vi "washinglogin.vi"() -> ()   [LabVIEW 2024]
uses:
  <vilib>/Utility/file.llb/Write Delimited Spreadsheet (string).vi
panel:
  in  "stop 9":bool
  in  "stop 4":bool
  out "bytes written 6":i32
  out "bytes written 5":i32
  in  "?":T1(tab)
  out "Validation":string
  in  "Edit":bool
  out "Boolean":bool
  in  "Delete":bool
  in  "Add":bool
  in  "Login":bool
  in  "Password":string
  in  "Username":string
  in  "?":bool
  in  "?":bool
  out "?":dbl(slide) scale=20.0..60.0
  out "?":dbl(slide) scale=20.0..60.0
  in  "?":enum16{"Soak", "Wash", "Rinse", "Spin"}(ring)
  in  "?":enum16{"Hot", "Default", "Cold"}(ring)
  in  "?":bool
  in  "?":enum16{"High", "Medium", "Low"}(ring)
  out "ON led":bool
  in  "?":bool
  out "?":dbl
  in  "?":dbl min=0.0 max=9999.0
  in  "?":string
  out "?":dbl
  in  "?":string
  in  "?":dbl min=0.0 max=9999.0
  in  "?":enum16{"Soak", "Wash", "Rinse", "Spin"}(ring)
  in  "?":bool
  in  "?":enum16{"High", "Medium", "Low"}(ring)
  out "?":dbl(slide) scale=20.0..60.0
  in  "?":enum16{"Hot", "Default", "Cold"}(ring)
  out "?":dbl(slide) scale=20.0..60.0
  out "?":bool
  in  "?":bool
  in  "?":bool
  in  "?":bool
  in  "?":string[][](table)
  in  "stop 8":bool
  out "bytes written 12":i32
  out "bytes written 11":i32
  in  "stop 7":bool
  out "bytes written 10":i32
  out "bytes written 9":i32
  in  "stop 6":bool
  out "bytes written 8":i32
  out "bytes written 7":i32
  in  "stop default true 8":bool
  in  "stop default true 7":bool
  in  "stop default true 6":bool
  in  "stop default true 5":bool
  in  "stop 5":bool
  in  "stop default true 4":bool
  out "bytes written":i32
  in  "stop":bool
  in  "stop default true":bool
  in  "stop default true 3":bool
  in  "stop default true 2":bool
  in  "stop 3":bool
  in  "stop 2":bool
  out "bytes written 4":i32
  out "bytes written 3":i32
  out "bytes written 2":i32
  # "OFF/ON"
  # "Water Level"
  # "Water Temperature"
  # "Select Mode"
  # "Current Operation"
  # "Set Operation Time"
  # "Timer"
  # "Water Level"
  # "Water Temperature"
  # "OFF/ON"
  # "ON led"
  # "Select Mode"
  # "Current Operation"
  # "Set Operation Time"
  # "Timer"
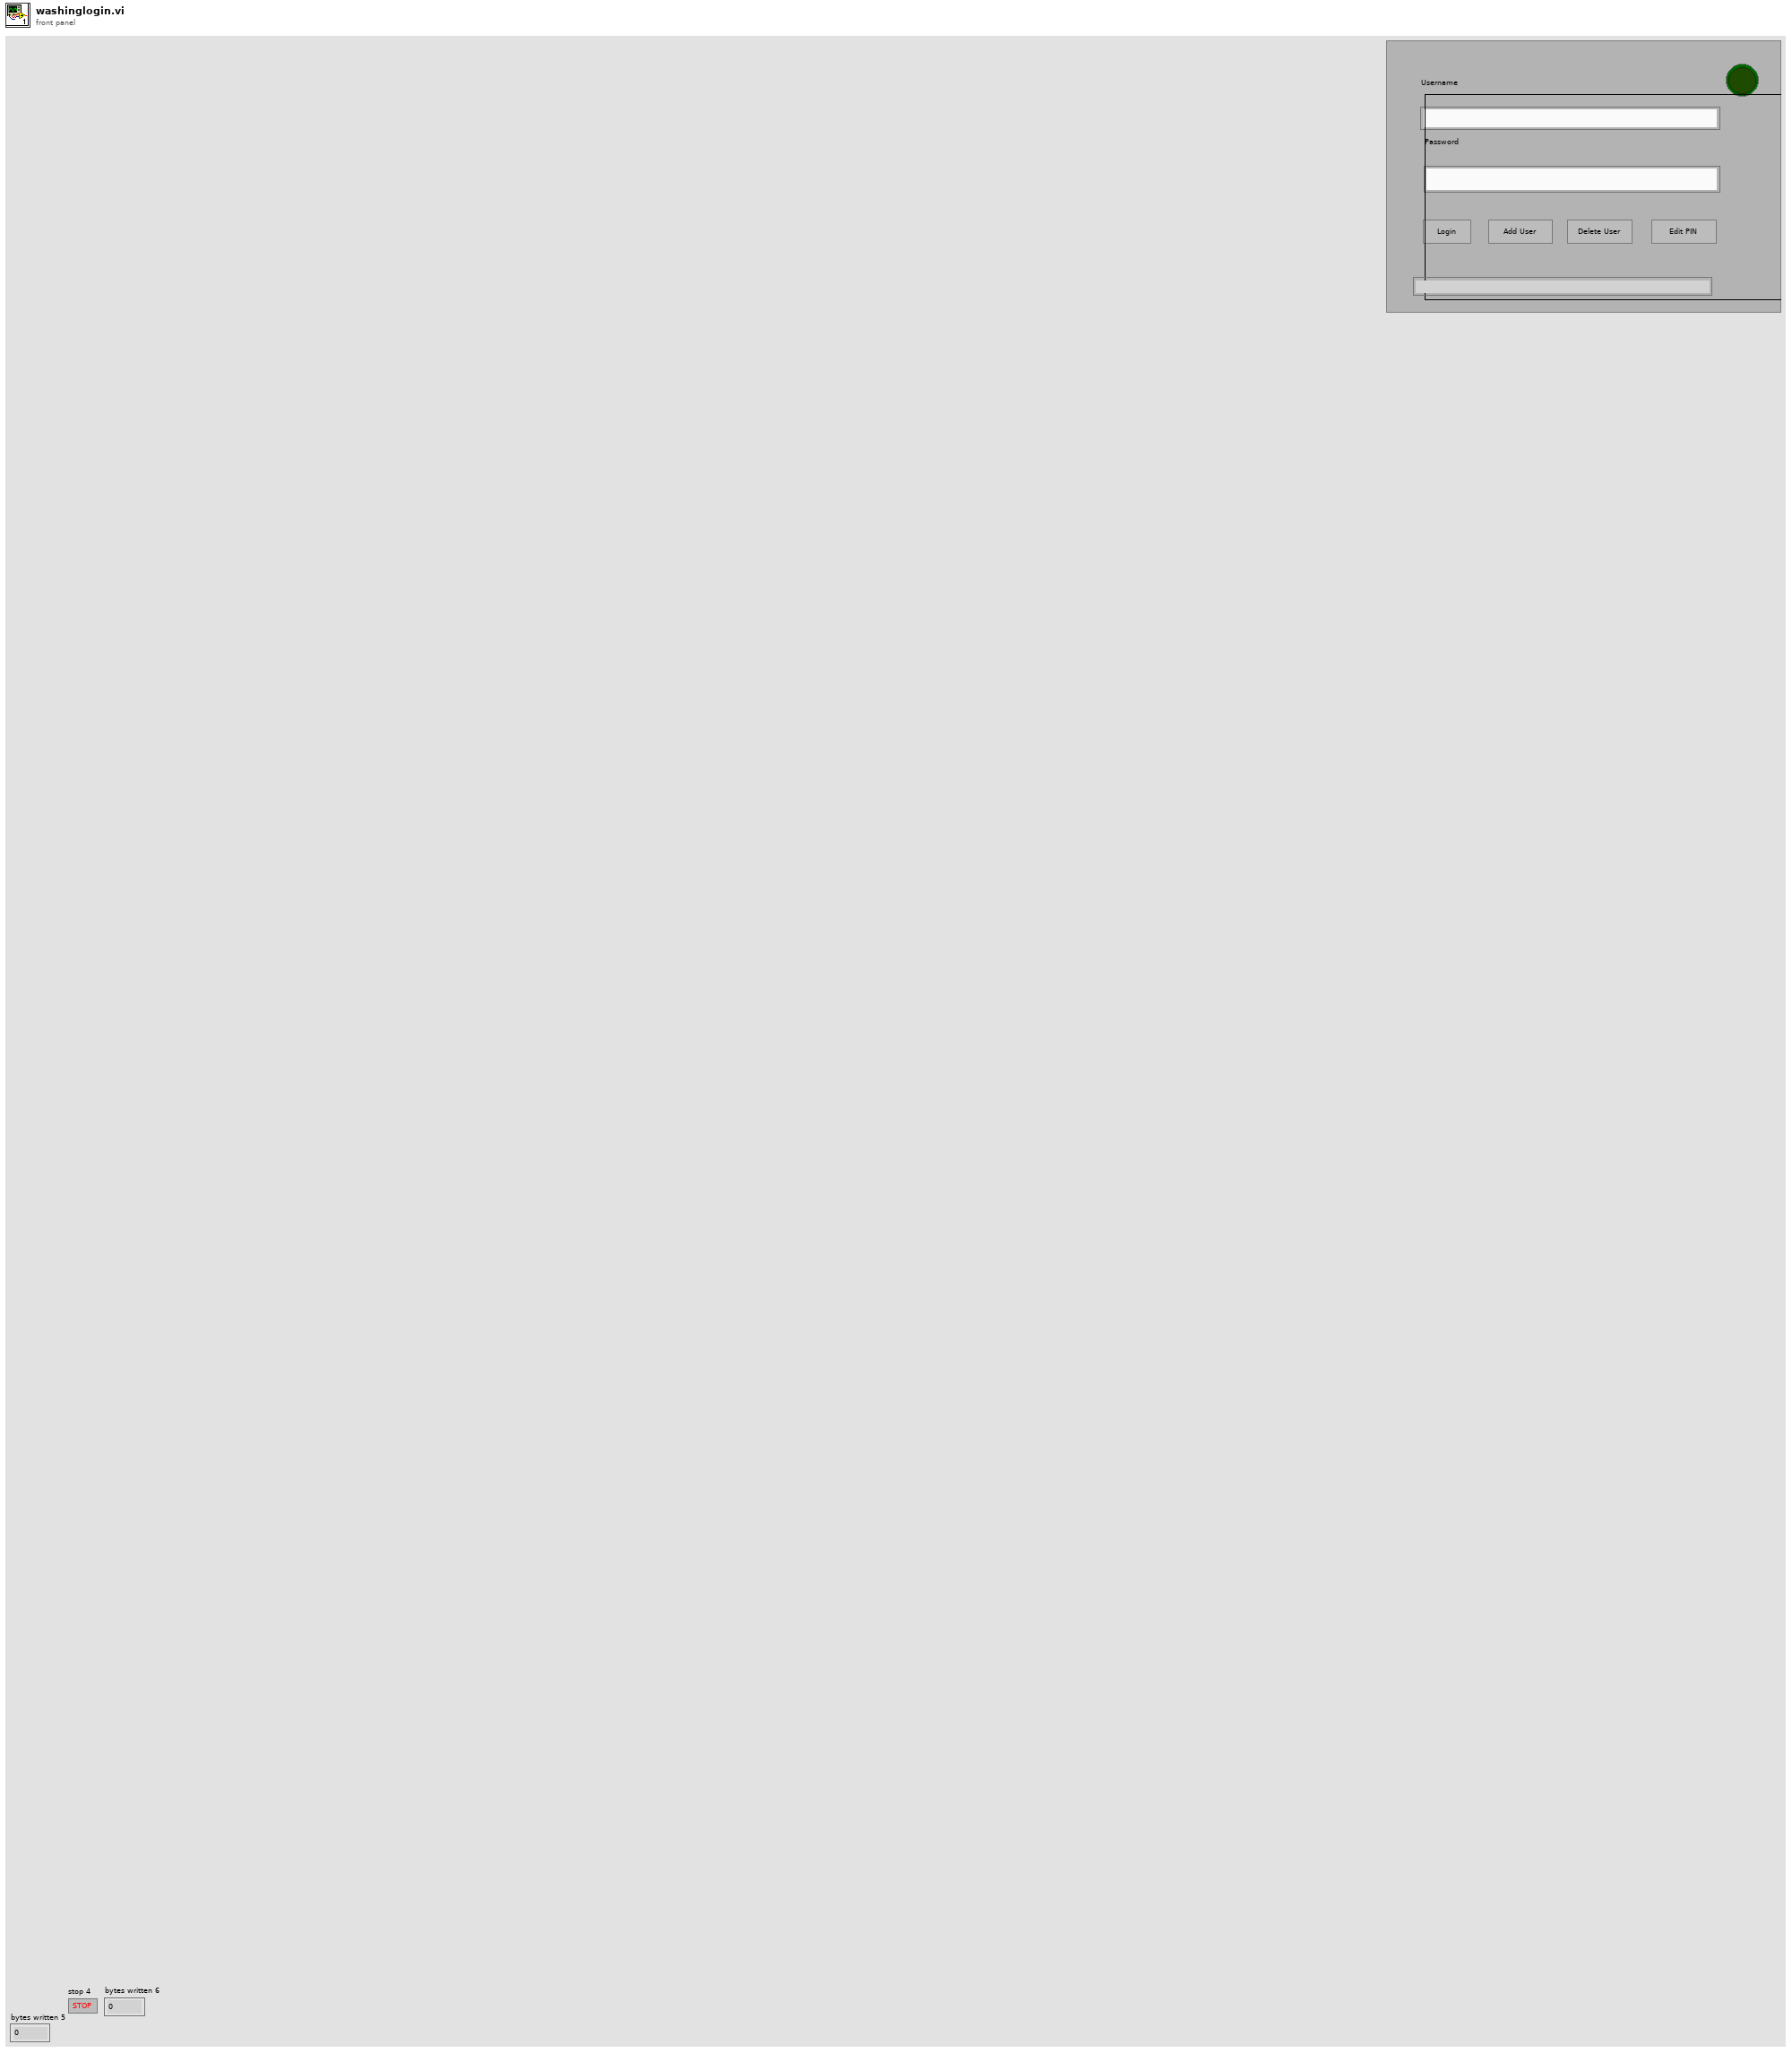
[diagram p1: front panel]
types:
  T1 = enum32{"Login", "Washing Machine 1", "Washing Machine 2", "usernamepassword"}
  T2 = enum32{"Login", "Washing Machine 1", "Washing Machine 2"}
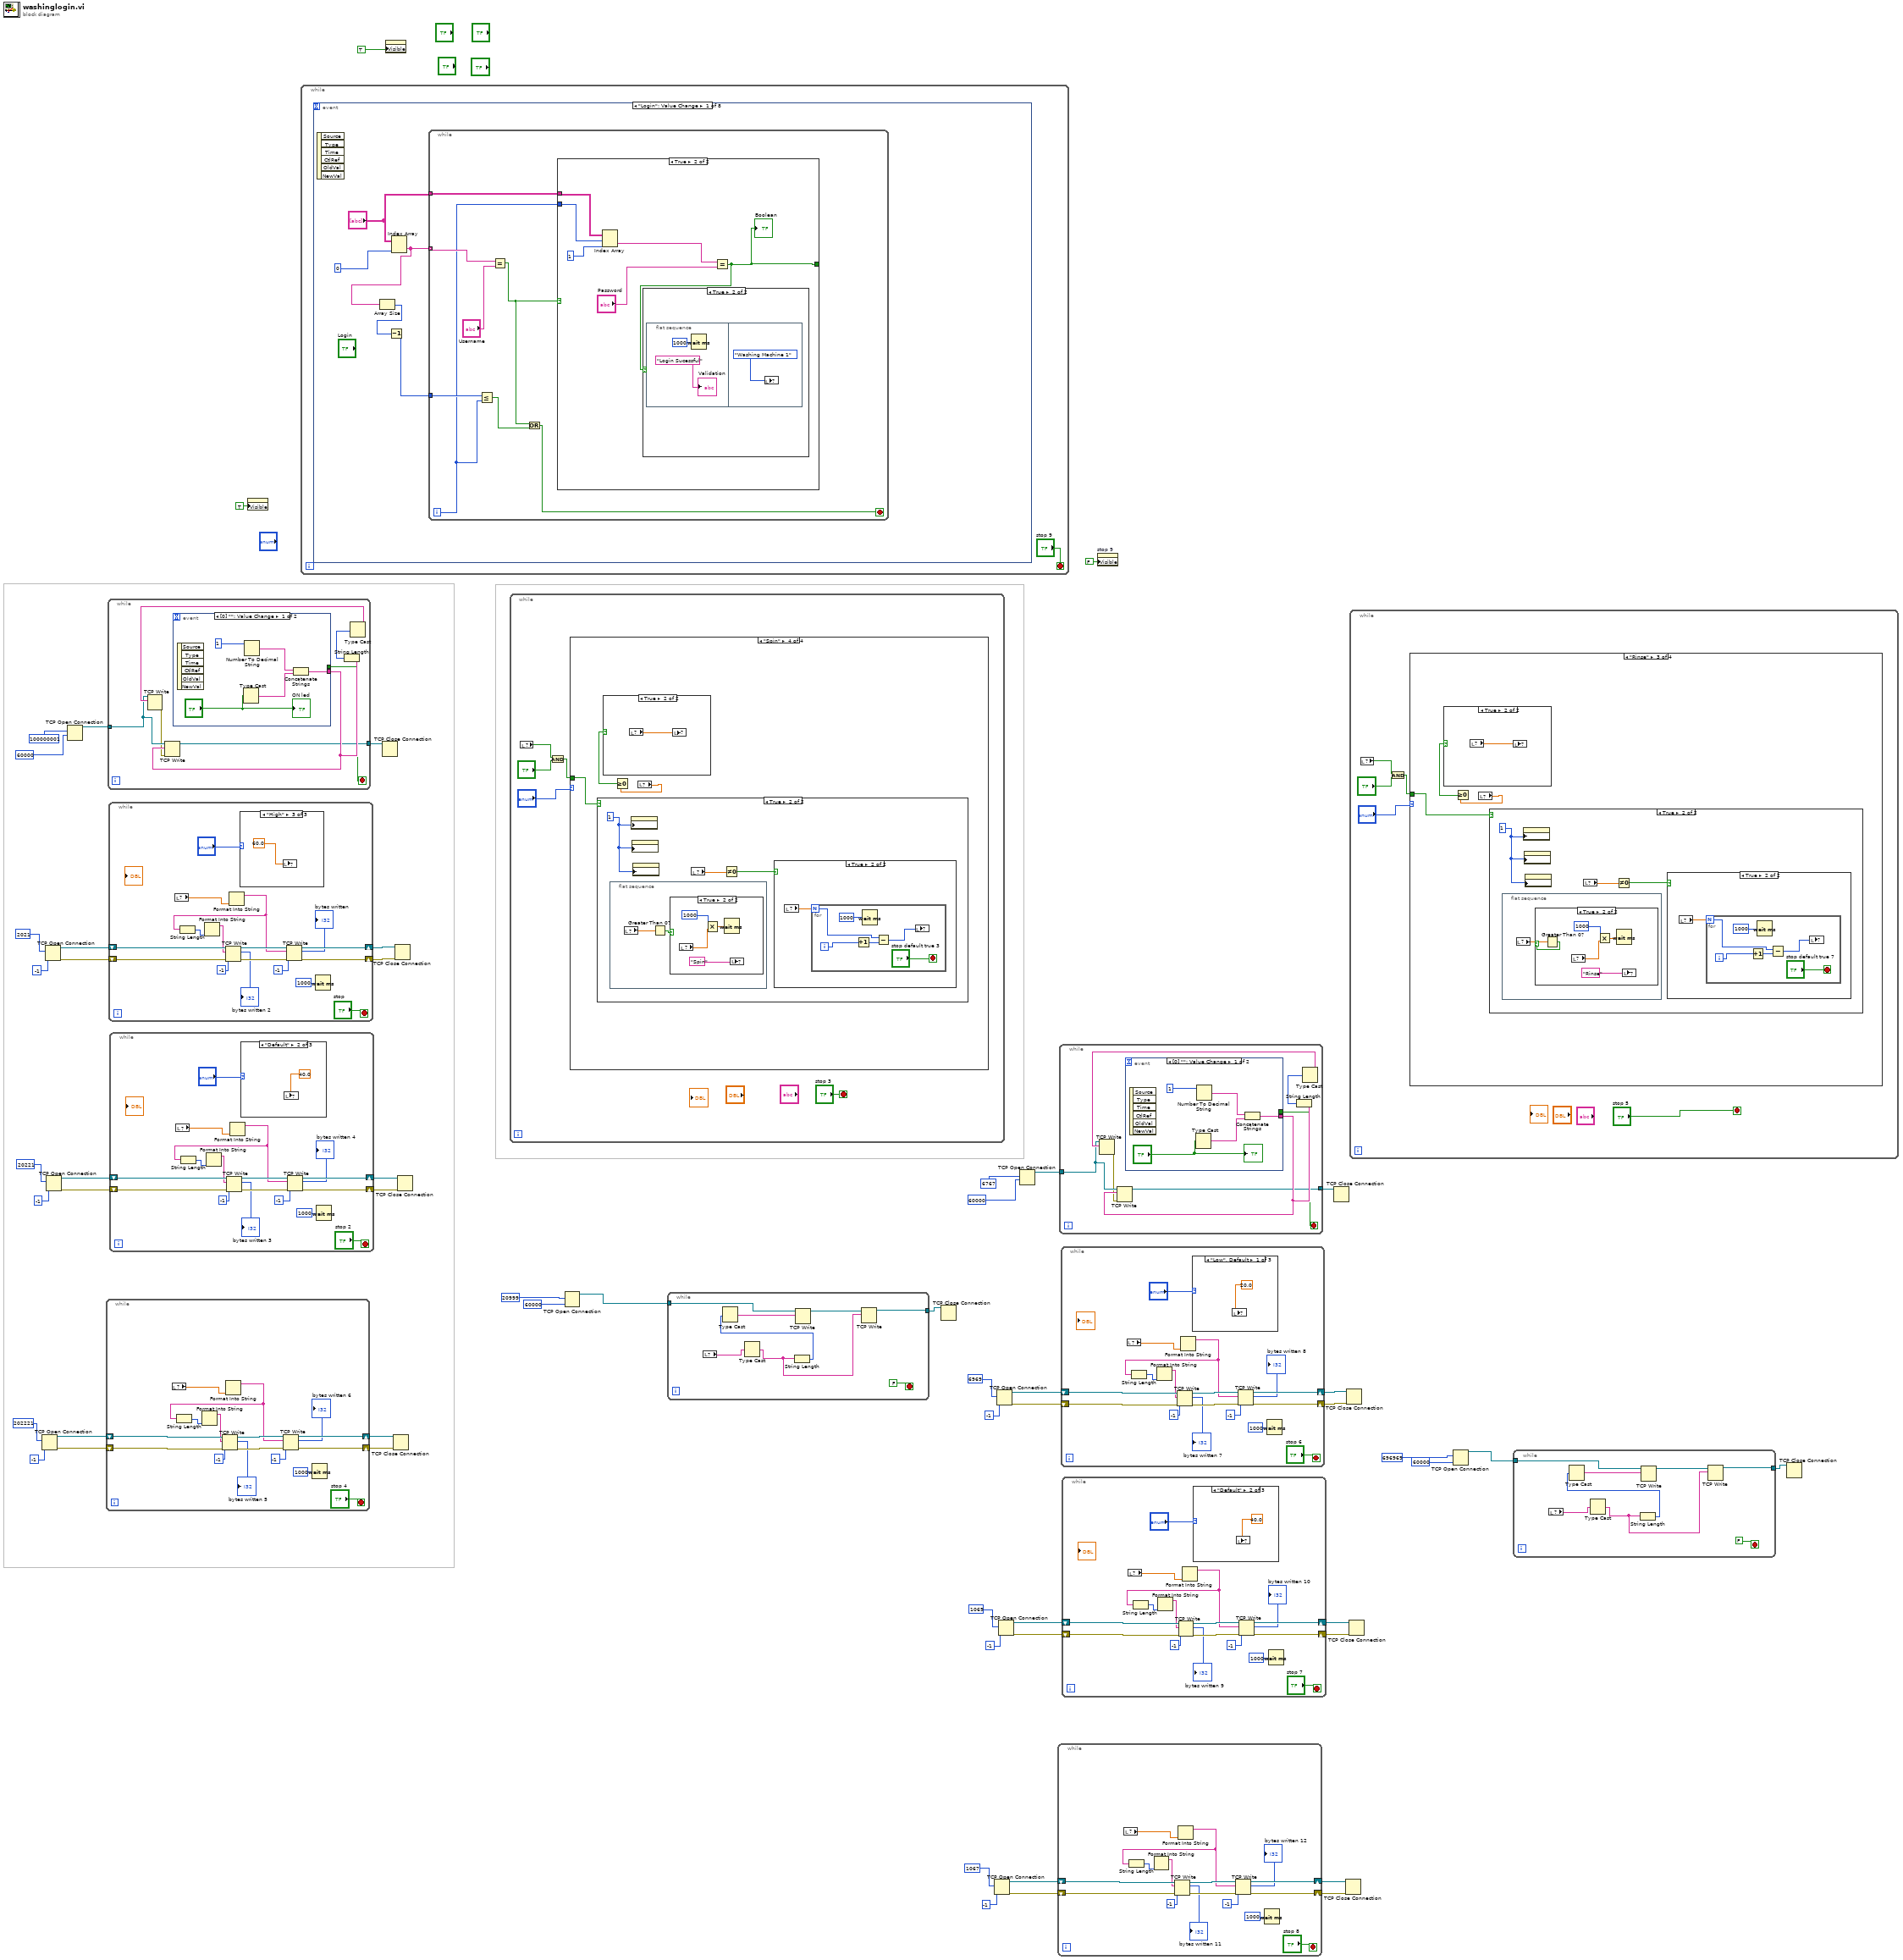
[diagram p0: block diagram]
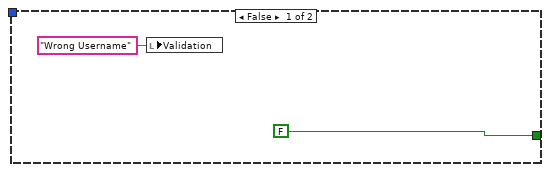
[diagram p2: hidden frame]
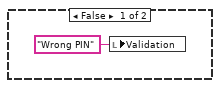
[diagram p3: hidden frame]
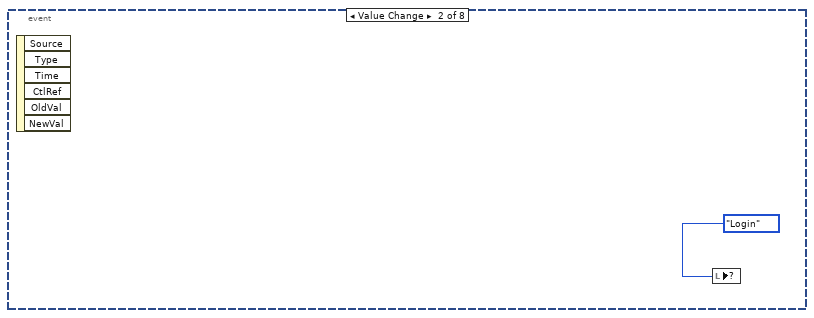
[diagram p4: hidden frame]
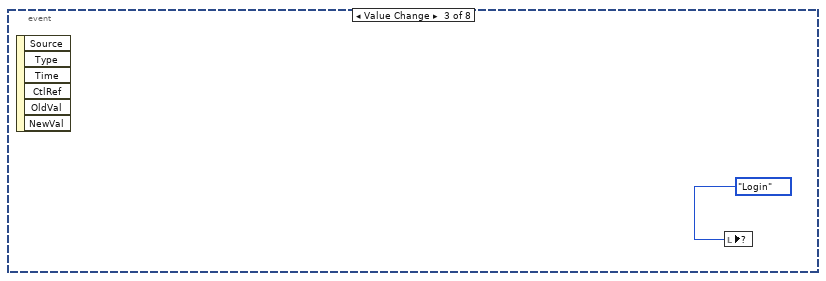
[diagram p5: hidden frame]
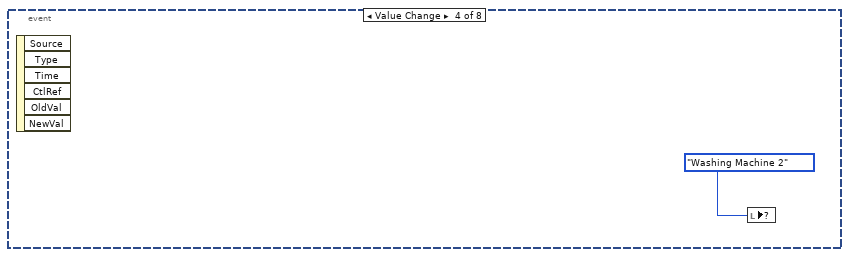
[diagram p6: hidden frame]
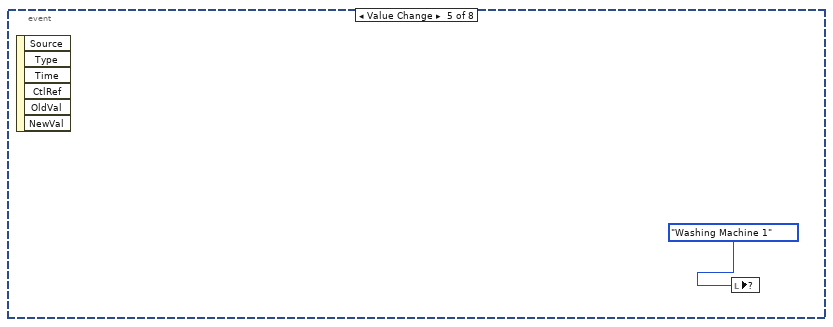
[diagram p7: hidden frame]
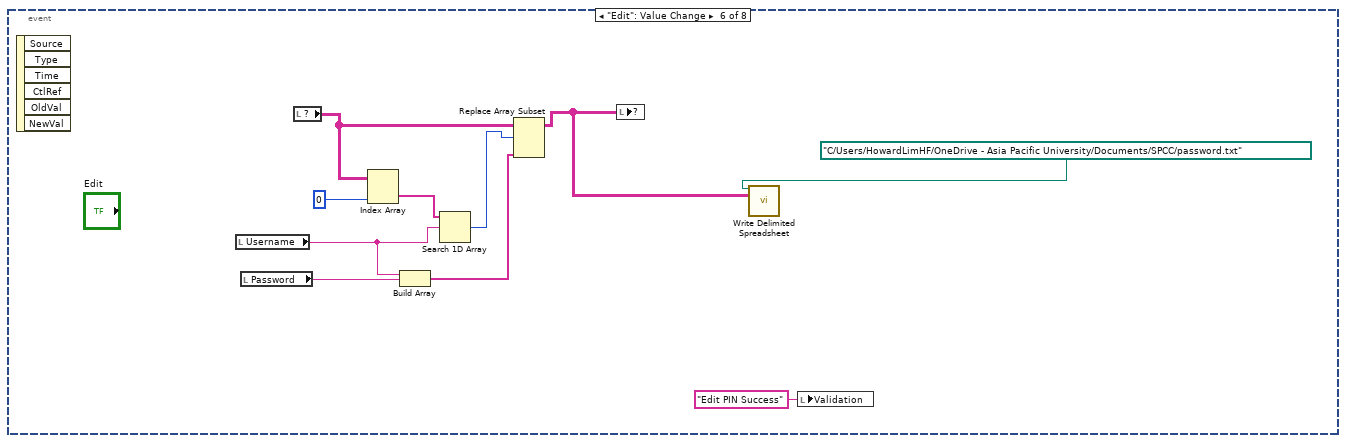
[diagram p8: hidden frame]
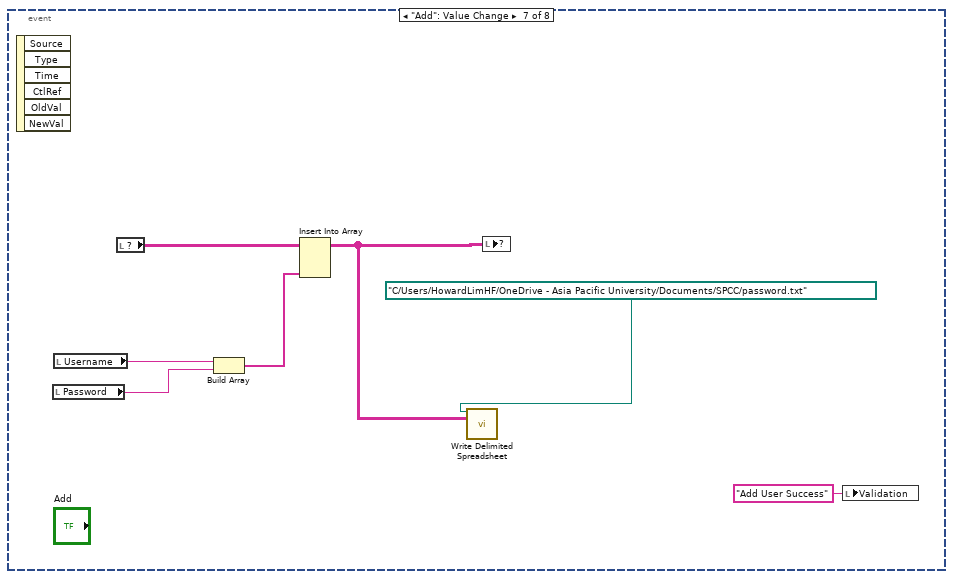
[diagram p9: hidden frame]
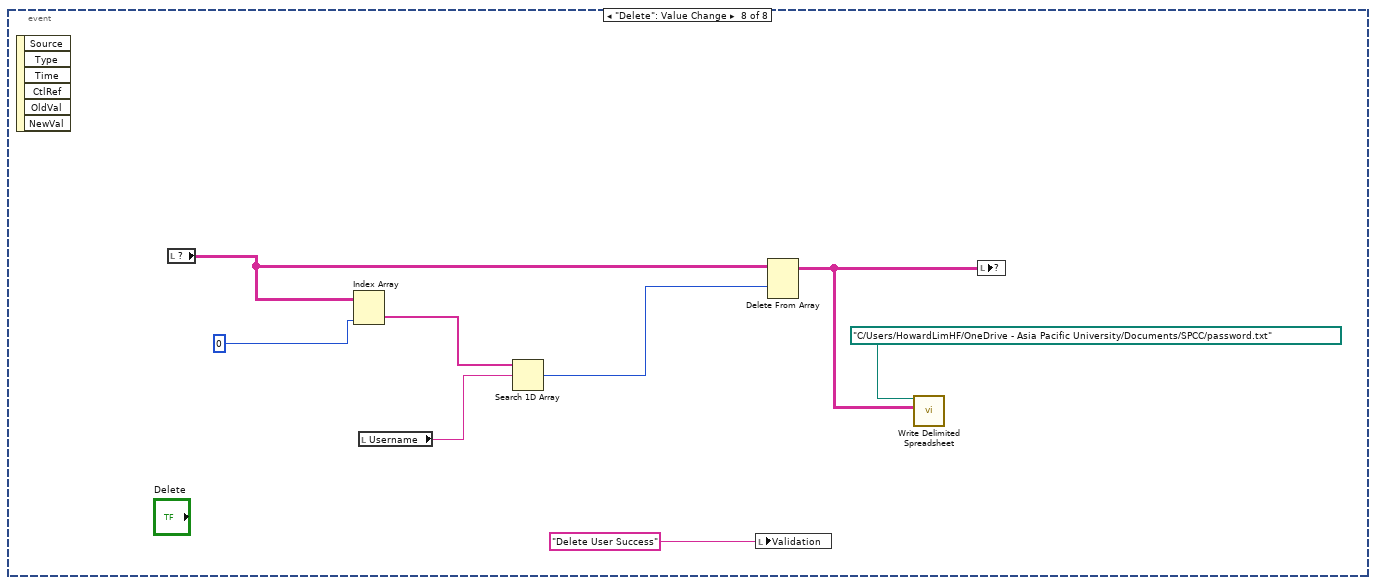
[diagram p10: hidden frame]
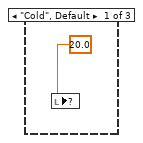
[diagram p11: hidden frame]
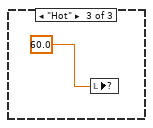
[diagram p12: hidden frame]
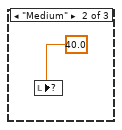
[diagram p13: hidden frame]
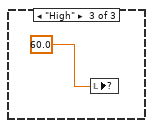
[diagram p14: hidden frame]
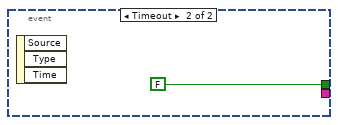
[diagram p15: hidden frame]
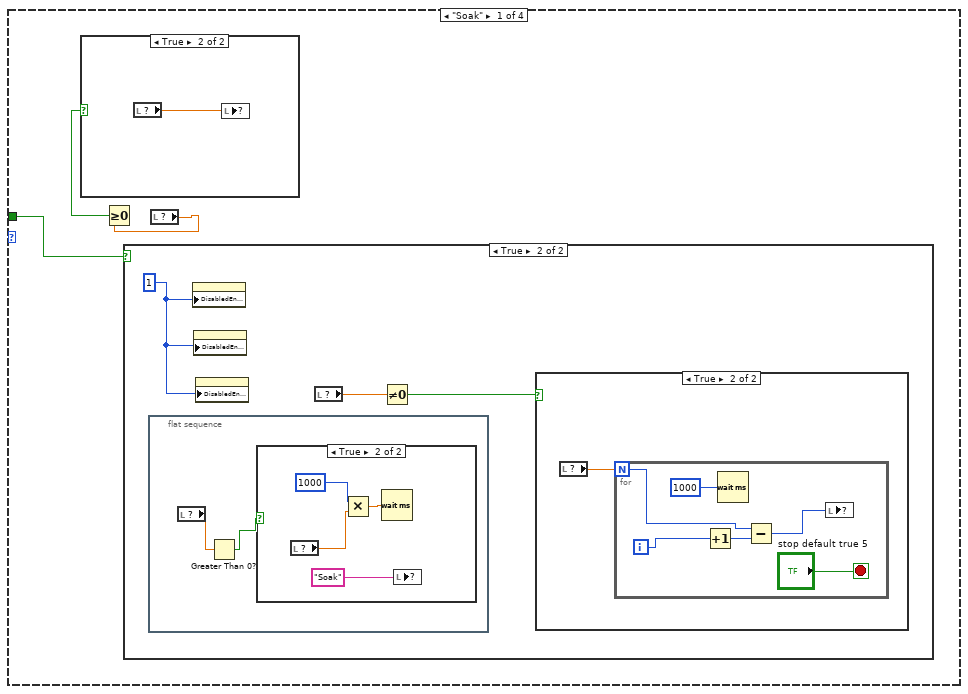
[diagram p16: hidden frame]
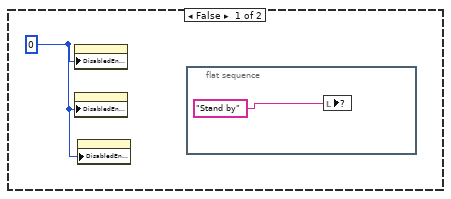
[diagram p18: hidden frame]
diagram:
  n1 = TCP Open Connection(remote port or service name=202221, timeout ms (60000)=-1) -> (connection ID=w35:refnum<k5>, error out=w37:errorcluster)  [unwired: 3 in]
  n2 = TCP Open Connection(remote port or service name=2021, timeout ms (60000)=-1) -> (connection ID=w47:refnum<k5>, error out=w49:errorcluster)  [unwired: 3 in]
  n3 = TCP Open Connection(remote port or service name=20221, timeout ms (60000)=-1) -> (connection ID=w41:refnum<k5>, error out=w43:errorcluster)  [unwired: 3 in]
  n4 = TCP Open Connection(remote port or service name=100000001, timeout ms (60000)=60000) -> (connection ID=w52:refnum<k5>)  [unwired: 3 in, 1 out]
  n5 = while {
    shift-right: [w69] -> w36
    shift-left: w35 -> [w71]
    shift-right: [w66] -> w38
    shift-left: w37 -> [w68]
    stop <- "stop 4" stop-if-true
    n6 = local read item#22() -> (w56:dbl)
    n7 = Format Into String(w56) -> (resulting string=w60:string)  [unwired: 3 in, 1 out]
    n8 = String Length(string=w60) -> (length=w59:i32)
    n9 = Format Into String(w59) -> (resulting string=w58:string)  [unwired: 3 in, 1 out]
    n10 = TCP Write(connection ID=w71, data in=w58, error in (no error)=w68, 9:-1 ("timeout ms (25000)")) -> (connection ID out=w70:refnum<k5>, bytes written=→"bytes written 5":i32, error out=w67:errorcluster)
    n11 = TCP Write(connection ID=w70, data in=w60, error in (no error)=w67, 9:-1 ("timeout ms (25000)")) -> (connection ID out=w69:refnum<k5>, bytes written=→"bytes written 6":i32, error out=w66:errorcluster)
    n12 = Wait (ms)(milliseconds to wait=u32 1000) -> ()  [unwired: 1 out]
  }
  n13 = while {
    tunnel: w52 -> [w76]
    tunnel: [w74] -> w51
    stop <- w73 stop-if-true
    n14 = event shown="[0] \"\": Value Change" {
      selector: _ -> [_ _]
      dyn-events: _ -> [_ _]
      timeout: _ -> [_ _]
      tunnel: [w80 _] -> w75
      tunnel: [_ FALSE] -> w73
      event Value Change {
        n15 = event-data() -> ()  [unwired: 1 in, 6 out]
        n16 = Type Cast(x="?") -> (*(type *) &x=w81:string)  [unwired: 1 in]
        n17 = Number To Decimal String(number=1) -> (decimal integer string=w82:string)  [unwired: 1 in]
        n18 = Concatenate Strings(w82, w81) -> (w80:string)
        "ON led" <- "?"
      }
      event Timeout {
        n19 = event-data() -> ()  [unwired: 1 in, 3 out]
      }
    }
    n20 = String Length(string=w75) -> (length=w78:i32)
    n21 = Type Cast(x=w78) -> (*(type *) &x=w77:string)  [unwired: 1 in]
    n22 = TCP Write(connection ID=w76, data in=w77) -> (error out=w72:errorcluster)  [unwired: 2 in, 2 out]
    n23 = TCP Write(connection ID=w76, data in=w75, error in (no error)=w72) -> (connection ID out=w74:refnum<k5>)  [unwired: 1 in, 2 out]
  }
  n24 = while {
    shift-right: [w99] -> w48
    shift-left: w47 -> [w101]
    shift-right: [w96] -> w50
    shift-left: w49 -> [w98]
    stop <- "stop" stop-if-true
    n25 = local read item#9() -> (w86:dbl)
    n26 = Format Into String(w86) -> (resulting string=w90:string)  [unwired: 3 in, 1 out]
    n27 = String Length(string=w90) -> (length=w89:i32)
    n28 = Format Into String(w89) -> (resulting string=w88:string)  [unwired: 3 in, 1 out]
    n29 = TCP Write(connection ID=w101, data in=w88, error in (no error)=w98, 9:-1 ("timeout ms (25000)")) -> (connection ID out=w100:refnum<k5>, bytes written=→"bytes written 2":i32, error out=w97:errorcluster)
    n30 = case shown="\"High\"" "?" {
      frame "Low", Default {
        n31 = local write item#9(20.0 ("Thermometer")) -> ()
      }
      frame "Medium" {
        n32 = local write item#9(40.0 ("Thermometer")) -> ()
      }
      frame "High" {
        n33 = local write item#9(60.0 ("Thermometer")) -> ()
      }
    }
    n34 = TCP Write(connection ID=w100, data in=w90, error in (no error)=w97, 9:-1 ("timeout ms (25000)")) -> (connection ID out=w99:refnum<k5>, bytes written=→"bytes written":i32, error out=w96:errorcluster)
    n35 = Wait (ms)(milliseconds to wait=u32 1000) -> ()  [unwired: 1 out]
  }
  n36 = while {
    shift-right: [w119] -> w42
    shift-left: w41 -> [w121]
    shift-right: [w116] -> w44
    shift-left: w43 -> [w118]
    stop <- "stop 2" stop-if-true
    n37 = local read item#16() -> (w106:dbl)
    n38 = Format Into String(w106) -> (resulting string=w110:string)  [unwired: 3 in, 1 out]
    n39 = String Length(string=w110) -> (length=w109:i32)
    n40 = Format Into String(w109) -> (resulting string=w108:string)  [unwired: 3 in, 1 out]
    n41 = TCP Write(connection ID=w121, data in=w108, error in (no error)=w118, 9:-1 ("timeout ms (25000)")) -> (connection ID out=w120:refnum<k5>, bytes written=→"bytes written 3":i32, error out=w117:errorcluster)
    n42 = case shown="\"Default\"" "?" {
      frame "Cold", Default {
        n43 = local write item#16(20.0 ("Thermometer")) -> ()
      }
      frame "Default" {
        n44 = local write item#16(40.0 ("Thermometer")) -> ()
      }
      frame "Hot" {
        n45 = local write item#16(60.0 ("Thermometer")) -> ()
      }
    }
    n46 = TCP Write(connection ID=w120, data in=w110, error in (no error)=w117, 9:-1 ("timeout ms (25000)")) -> (connection ID out=w119:refnum<k5>, bytes written=→"bytes written 4":i32, error out=w116:errorcluster)
    n47 = Wait (ms)(milliseconds to wait=u32 1000) -> ()  [unwired: 1 out]
  }
  n48 = property class="TabCtl (strict)"("Visible"=TRUE) -> ()  [unwired: 2 in, 2 out]
  n49 = while {
    stop <- "stop 9" stop-if-true
    n50 = event shown="[0] \"Login\": Value Change" {
      selector: _ -> [_ _ _ _ _ _ _ _]
      dyn-events: _ -> [_ _ _ _ _ _ _ _]
      timeout: _ -> [_ _ _ _ _ _ _ _]
      event "Login": Value Change {
        n51 = event-data() -> ()  [unwired: 1 in, 6 out]
        n52 = Index Array "Index Array"(array="?", index (col)=0) -> (element=w128:string[])  [unwired: 1 in]
        n53 = Array Size(array=w128) -> (size(s)=w127:i32)
        n54 = Decrement(x=w127) -> (x-1=w126:i32)
        n55 = while {
          tunnel: "?" -> [w137]
          tunnel: w128 -> [w136] mode=indexing
          tunnel: w126 -> [w135]
          i -> [w134]
          stop <- w131 stop-if-true
          n56 = Less Or Equal?(x=w135, y=w134) -> (x <= y?=w132:bool)
          n57 = Equal?(x=w136, y="Username") -> (x = y?=w133:bool)
          n58 = Or(x=w133, y=w132) -> (x .or. y?=w131:bool)
          n59 = case shown="True" w133 {
            tunnel: w137 -> [_ w146]
            tunnel: w134 -> [_ w145]
            tunnel: [FALSE w141] -> _
            frame False {
              n60 = local write "Validation"("Wrong Username" ("Validation")) -> ()
            }
            frame True {
              n61 = Index Array "Index Array"(array=w146, index (row)=w145, index (col)=1) -> (element=w143:string)
              n62 = Equal?(x=w143, y="Password") -> (x = y?=w141:bool)
              "Boolean" <- w141
              n63 = case shown="True" w141 {
                frame False {
                  n64 = local write "Validation"("Wrong PIN" ("Validation")) -> ()
                }
                frame True {
                  n65 = flat-sequence {
                    frame #0 {
                      n66 = Wait (ms)(milliseconds to wait=u32 1000) -> ()  [unwired: 1 out]
                      "Validation" <- "Login Sucessful" ("Validation")
                    }
                    frame #1 {
                      n67 = local write item#?(T2."Washing Machine 1" ("Tab Control")) -> ()
                    }
                  }
                }
              }
            }
          }
        }
      }
      event Value Change {
        n68 = event-data() -> ()  [unwired: 1 in, 6 out]
        n69 = local write item#?(T2."Login" ("Tab Control")) -> ()
      }
      event Value Change {
        n70 = event-data() -> ()  [unwired: 1 in, 6 out]
        n71 = local write item#?(T2."Login" ("Tab Control")) -> ()
      }
      event Value Change {
        n72 = event-data() -> ()  [unwired: 1 in, 6 out]
        n73 = local write item#?(T2."Washing Machine 2" ("Tab Control")) -> ()
      }
      event Value Change {
        n74 = event-data() -> ()  [unwired: 1 in, 6 out]
        n75 = local write item#?(T2."Washing Machine 1" ("Tab Control")) -> ()
      }
      event "Edit": Value Change {
        n76 = event-data() -> ()  [unwired: 1 in, 6 out]
        n77 = local read "Username"() -> (w159:string)
        n78 = local read "Password"() -> (w160:string)
        n79 = local read item#7() -> (w156:string[][])
        n80 = Index Array(array=w156, index (col)=0 ("disabled index (col)")) -> (element=w161:string[])  [unwired: 1 in]
        n81 = Build Array(w159, w160) -> (w158:string[])
        n82 = Search 1D Array(1D array=w161, element=w159) -> (index of element=w157:i32)  [unwired: 1 in]
        n83 = Replace Array Subset(array=w156, new element=w158, index (row)=w157) -> (w155:string[][])  [unwired: 1 in]
        n84 = local write item#7(w155) -> ()
        n85 = call-poly <vilib>:"Write Delimited Spreadsheet.vi"("file path (dialog if empty)"=path "C:/Users/HowardLimHF/OneDrive - Asia Pacific University/Documents/SPCC/password.txt", "2D data"=w155) -> ()  [unwired: 12 in, 2 out]
        n86 = local write "Validation"("Edit PIN Success" ("Validation")) -> ()
      }
      event "Add": Value Change {
        n87 = event-data() -> ()  [unwired: 1 in, 6 out]
        n88 = local read "Password"() -> (w170:string)
        n89 = local read "Username"() -> (w171:string)
        n90 = local read item#7() -> (w169:string[][])
        n91 = Build Array "Build Array"(w171, w170) -> (w168:string[])
        n92 = Insert Into Array "Insert Into Array"(array=w169, new element=w168) -> (w167:string[][])  [unwired: 2 in]
        n93 = call-poly <vilib>:"Write Delimited Spreadsheet.vi"("file path (dialog if empty)"=path "C:/Users/HowardLimHF/OneDrive - Asia Pacific University/Documents/SPCC/password.txt", "2D data"=w167) -> ()  [unwired: 12 in, 2 out]
        n94 = local write item#7(w167) -> ()
        n95 = local write "Validation"("Add User Success" ("Validation")) -> ()
      }
      event "Delete": Value Change {
        n96 = event-data() -> ()  [unwired: 1 in, 6 out]
        n97 = local read item#7() -> (w175:string[][])
        n98 = Index Array "Index Array"(array=w175, index (col)=0) -> (element=w178:string[])  [unwired: 1 in]
        n99 = local read "Username"() -> (w177:string)
        n100 = Search 1D Array(1D array=w178, element=w177) -> (index of element=w176:i32)  [unwired: 1 in]
        n101 = local write "Validation"("Delete User Success" ("Validation")) -> ()
        n102 = Delete From Array "Delete From Array"(array=w175, index (row)=w176) -> (array with subset deleted=w174:string[][])  [unwired: 2 in, 1 out]
        n103 = call-poly <vilib>:"Write Delimited Spreadsheet.vi"("file path (dialog if empty)"=path "C:/Users/HowardLimHF/OneDrive - Asia Pacific University/Documents/SPCC/password.txt", "2D data"=w174) -> ()  [unwired: 12 in, 2 out]
        n104 = local write item#7(w174) -> ()
      }
    }
  }
  n105 = TCP Close Connection(connection ID=w51) -> ()  [unwired: 2 in, 2 out]
  n106 = property class="Tbl (strict)"("Visible"=TRUE) -> ()  [unwired: 2 in, 2 out]
  n107 = TCP Close Connection(connection ID=w36, error in (no error)=w38) -> ()  [unwired: 1 in, 2 out]
  n108 = TCP Close Connection(connection ID=w48, error in (no error)=w50) -> ()  [unwired: 1 in, 2 out]
  n109 = TCP Close Connection(connection ID=w42, error in (no error)=w44) -> ()  [unwired: 1 in, 2 out]
  n110 = while {
    stop <- "stop 3" stop-if-true
    n111 = local read item#8() -> (w184:bool)
    n112 = And(x=w184, y="?") -> (x .and. y?=w180:bool)
    n113 = case shown="\"Spin\"" "?" {
      tunnel: w180 -> [w185 w207 w229 w251]
      frame "Soak" {
        n114 = case shown="True" w185 {
          frame False {
            w189 = 0
            n115 = property class="Enum (strict)"("DisabledEnum"=w189) -> ()  [unwired: 2 in, 2 out]
            n116 = property class="Slide (strict)"("DisabledEnum"=w189) -> ()  [unwired: 2 in, 2 out]
            n117 = property class="Slide (strict)"("DisabledEnum"=w189) -> ()  [unwired: 2 in, 2 out]
            n118 = flat-sequence {
              frame #0 {
                n119 = local write item#24("Stand by") -> ()
              }
            }
          }
          frame True {
            w193 = 1
            n120 = flat-sequence {
              frame #0 {
                n121 = local read item#22() -> (w195:dbl)
                n122 = Greater Than 0?(x=w195) -> (x > 0?=w194:bool)
                n123 = case shown="True" w194 {
                  frame False {
                  }
                  frame True {
                    n124 = local read item#22() -> (w198:dbl)
                    n125 = Multiply(x=1000, y=w198) -> (x*y=w197:dbl)
                    n126 = Wait (ms)(milliseconds to wait=w197) -> ()  [unwired: 1 out]
                    n127 = local write item#24("Soak") -> ()
                  }
                }
              }
            }
            n128 = property class="Enum (strict)"("DisabledEnum"=w193) -> ()  [unwired: 2 in, 2 out]
            n129 = property class="Slide (strict)"("DisabledEnum"=w193) -> ()  [unwired: 2 in, 2 out]
            n130 = property class="Slide (strict)"("DisabledEnum"=w193) -> ()  [unwired: 2 in, 2 out]
            n131 = local read item#22() -> (w192:dbl)
            n132 = Not Equal To 0?(x=w192) -> (x != 0?=w191:bool)
            n133 = case shown="True" w191 {
              frame False {
              }
              frame True {
                n134 = local read item#22() -> (w200:dbl)
                n135 = for {
                  N: w200 -> [w206]
                  i -> [w202]
                  stop <- "stop default true 4" stop-if-true
                  n136 = Increment(x=w202) -> (x+1=w205:i32)
                  n137 = Wait (ms)(milliseconds to wait=u32 1000) -> ()  [unwired: 1 out]
                  n138 = Subtract(x=w206, y=w205) -> (x-y=w203:i32)
                  n139 = local write item#22(w203) -> ()
                }
              }
            }
          }
        }
        n140 = local read item#22() -> (w187:dbl)
        n141 = Greater Or Equal To 0?(x=w187) -> (x >= 0?=w186:bool)
        n142 = case shown="True" w186 {
          frame False {
          }
          frame True {
            n143 = local read item#23() -> (w188:dbl)
            n144 = local write item#22(w188) -> ()
          }
        }
      }
      frame "Wash" {
        n145 = case shown="True" w207 {
          frame False {
            w211 = 0
            n146 = property class="Enum (strict)"("DisabledEnum"=w211) -> ()  [unwired: 2 in, 2 out]
            n147 = property class="Slide (strict)"("DisabledEnum"=w211) -> ()  [unwired: 2 in, 2 out]
            n148 = property class="Slide (strict)"("DisabledEnum"=w211) -> ()  [unwired: 2 in, 2 out]
            n149 = flat-sequence {
              frame #0 {
                n150 = local write item#24("Stand by") -> ()
              }
            }
          }
          frame True {
            w215 = 1
            n151 = flat-sequence {
              frame #0 {
                n152 = local read item#22() -> (w217:dbl)
                n153 = Greater Than 0?(x=w217) -> (x > 0?=w216:bool)
                n154 = case shown="True" w216 {
                  frame False {
                  }
                  frame True {
                    n155 = local read item#22() -> (w220:dbl)
                    n156 = Multiply(x=1000, y=w220) -> (x*y=w219:dbl)
                    n157 = Wait (ms)(milliseconds to wait=w219) -> ()  [unwired: 1 out]
                    n158 = local write item#24("Wash") -> ()
                  }
                }
              }
            }
            n159 = property class="Enum (strict)"("DisabledEnum"=w215) -> ()  [unwired: 2 in, 2 out]
            n160 = property class="Slide (strict)"("DisabledEnum"=w215) -> ()  [unwired: 2 in, 2 out]
            n161 = property class="Slide (strict)"("DisabledEnum"=w215) -> ()  [unwired: 2 in, 2 out]
            n162 = local read item#22() -> (w214:dbl)
            n163 = Not Equal To 0?(x=w214) -> (x != 0?=w213:bool)
            n164 = case shown="True" w213 {
              frame False {
              }
              frame True {
                n165 = local read item#22() -> (w222:dbl)
                n166 = for {
                  N: w222 -> [w228]
                  i -> [w224]
                  stop <- "stop default true" stop-if-true
                  n167 = Increment(x=w224) -> (x+1=w227:i32)
                  n168 = Wait (ms)(milliseconds to wait=u32 1000) -> ()  [unwired: 1 out]
                  n169 = Subtract(x=w228, y=w227) -> (x-y=w225:i32)
                  n170 = local write item#22(w225) -> ()
                }
              }
            }
          }
        }
        n171 = local read item#22() -> (w209:dbl)
        n172 = Equal To 0?(x=w209) -> (x = 0?=w208:bool)
        n173 = case shown="True" w208 {
          frame False {
          }
          frame True {
            n174 = local read item#23() -> (w210:dbl)
            n175 = local write item#22(w210) -> ()
          }
        }
      }
      frame "Rinse" {
        n176 = case shown="True" w229 {
          frame False {
            w233 = 0
            n177 = property class="Slide (strict)"("DisabledEnum"=w233) -> ()  [unwired: 2 in, 2 out]
            n178 = property class="Slide (strict)"("DisabledEnum"=w233) -> ()  [unwired: 2 in, 2 out]
            n179 = property class="Enum (strict)"("DisabledEnum"=w233) -> ()  [unwired: 2 in, 2 out]
            n180 = flat-sequence {
              frame #0 {
                n181 = local write item#24("Stand by") -> ()
              }
            }
          }
          frame True {
            w237 = 1
            n182 = flat-sequence {
              frame #0 {
                n183 = local read item#22() -> (w239:dbl)
                n184 = Greater Than 0?(x=w239) -> (x > 0?=w238:bool)
                n185 = case shown="True" w238 {
                  frame False {
                  }
                  frame True {
                    n186 = local read item#22() -> (w242:dbl)
                    n187 = Multiply(x=1000, y=w242) -> (x*y=w241:dbl)
                    n188 = Wait (ms)(milliseconds to wait=w241) -> ()  [unwired: 1 out]
                    n189 = local write item#24("Rinse") -> ()
                  }
                }
              }
            }
            n190 = property class="Enum (strict)"("DisabledEnum"=w237) -> ()  [unwired: 2 in, 2 out]
            n191 = property class="Slide (strict)"("DisabledEnum"=w237) -> ()  [unwired: 2 in, 2 out]
            n192 = property class="Slide (strict)"("DisabledEnum"=w237) -> ()  [unwired: 2 in, 2 out]
            n193 = local read item#22() -> (w236:dbl)
            n194 = Not Equal To 0?(x=w236) -> (x != 0?=w235:bool)
            n195 = case shown="True" w235 {
              frame False {
              }
              frame True {
                n196 = local read item#22() -> (w244:dbl)
                n197 = for {
                  N: w244 -> [w250]
                  i -> [w246]
                  stop <- "stop default true 2" stop-if-true
                  n198 = Increment(x=w246) -> (x+1=w249:i32)
                  n199 = Wait (ms)(milliseconds to wait=u32 1000) -> ()  [unwired: 1 out]
                  n200 = Subtract(x=w250, y=w249) -> (x-y=w247:i32)
                  n201 = local write item#22(w247) -> ()
                }
              }
            }
          }
        }
        n202 = local read item#22() -> (w231:dbl)
        n203 = Greater Or Equal To 0?(x=w231) -> (x >= 0?=w230:bool)
        n204 = case shown="True" w230 {
          frame False {
          }
          frame True {
            n205 = local read item#23() -> (w232:dbl)
            n206 = local write item#22(w232) -> ()
          }
        }
      }
      frame "Spin" {
        n207 = case shown="True" w251 {
          frame False {
            w255 = 0
            n208 = property class="Enum (strict)"("DisabledEnum"=w255) -> ()  [unwired: 2 in, 2 out]
            n209 = property class="Slide (strict)"("DisabledEnum"=w255) -> ()  [unwired: 2 in, 2 out]
            n210 = property class="Slide (strict)"("DisabledEnum"=w255) -> ()  [unwired: 2 in, 2 out]
            n211 = flat-sequence {
              frame #0 {
                n212 = local write item#24("Stand by") -> ()
              }
            }
          }
          frame True {
            w259 = 1
            n213 = flat-sequence {
              frame #0 {
                n214 = local read item#22() -> (w261:dbl)
                n215 = Greater Than 0?(x=w261) -> (x > 0?=w260:bool)
                n216 = case shown="True" w260 {
                  frame False {
                  }
                  frame True {
                    n217 = local read item#22() -> (w264:dbl)
                    n218 = Multiply(x=1000, y=w264) -> (x*y=w263:dbl)
                    n219 = Wait (ms)(milliseconds to wait=w263) -> ()  [unwired: 1 out]
                    n220 = local write item#24("Spin") -> ()
                  }
                }
              }
            }
            n221 = property class="Enum (strict)"("DisabledEnum"=w259) -> ()  [unwired: 2 in, 2 out]
            n222 = property class="Slide (strict)"("DisabledEnum"=w259) -> ()  [unwired: 2 in, 2 out]
            n223 = property class="Slide (strict)"("DisabledEnum"=w259) -> ()  [unwired: 2 in, 2 out]
            n224 = local read item#22() -> (w258:dbl)
            n225 = Not Equal To 0?(x=w258) -> (x != 0?=w257:bool)
            n226 = case shown="True" w257 {
              frame False {
              }
              frame True {
                n227 = local read item#22() -> (w266:dbl)
                n228 = for {
                  N: w266 -> [w272]
                  i -> [w268]
                  stop <- "stop default true 3" stop-if-true
                  n229 = Increment(x=w268) -> (x+1=w271:i32)
                  n230 = Wait (ms)(milliseconds to wait=u32 1000) -> ()  [unwired: 1 out]
                  n231 = Subtract(x=w272, y=w271) -> (x-y=w269:i32)
                  n232 = local write item#22(w269) -> ()
                }
              }
            }
          }
        }
        n233 = local read item#22() -> (w252:dbl)
        n234 = Greater Or Equal To 0?(x=w252) -> (x >= 0?=w253:bool)
        n235 = case shown="True" w253 {
          frame False {
          }
          frame True {
            n236 = local read item#23() -> (w254:dbl)
            n237 = local write item#22(w254) -> ()
          }
        }
      }
    }
  }
  n238 = TCP Open Connection(remote port or service name=20999, timeout ms (60000)=60000) -> (connection ID=w29:refnum<k5>)  [unwired: 3 in, 1 out]
  n239 = while {
    tunnel: [w276] -> w32
    tunnel: w29 -> [w275]
    stop <- FALSE stop-if-true
    n240 = local read item#24() -> (w274:string)
    n241 = Type Cast(x=w274) -> (*(type *) &x=w273:string)  [unwired: 1 in]
    n242 = String Length(string=w273) -> (length=w280:i32)
    n243 = Type Cast(x=w280) -> (*(type *) &x=w279:string)  [unwired: 1 in]
    n244 = TCP Write(connection ID=w275, data in=w279) -> (connection ID out=w277:refnum<k5>)  [unwired: 2 in, 2 out]
    n245 = TCP Write(connection ID=w277, data in=w273) -> (connection ID out=w276:refnum<k5>)  [unwired: 2 in, 2 out]
  }
  n246 = TCP Close Connection(connection ID=w32) -> ()  [unwired: 2 in, 2 out]
  n247 = TCP Open Connection(remote port or service name=1067, timeout ms (60000)=-1) -> (connection ID=w9:refnum<k5>, error out=w11:errorcluster)  [unwired: 3 in]
  n248 = TCP Open Connection(remote port or service name=6969, timeout ms (60000)=-1) -> (connection ID=w21:refnum<k5>, error out=w23:errorcluster)  [unwired: 3 in]
  n249 = TCP Open Connection(remote port or service name=1069, timeout ms (60000)=-1) -> (connection ID=w15:refnum<k5>, error out=w17:errorcluster)  [unwired: 3 in]
  n250 = TCP Open Connection(remote port or service name=6767, timeout ms (60000)=60000) -> (connection ID=w26:refnum<k5>)  [unwired: 3 in, 1 out]
  n251 = while {
    shift-right: [w294] -> w10
    shift-left: w9 -> [w296]
    shift-right: [w291] -> w12
    shift-left: w11 -> [w293]
    stop <- "stop 8" stop-if-true
    n252 = local read item#34() -> (w281:dbl)
    n253 = Format Into String(w281) -> (resulting string=w285:string)  [unwired: 3 in, 1 out]
    n254 = String Length(string=w285) -> (length=w284:i32)
    n255 = Format Into String(w284) -> (resulting string=w283:string)  [unwired: 3 in, 1 out]
    n256 = TCP Write(connection ID=w296, data in=w283, error in (no error)=w293, 9:-1 ("timeout ms (25000)")) -> (connection ID out=w295:refnum<k5>, bytes written=→"bytes written 11":i32, error out=w292:errorcluster)
    n257 = TCP Write(connection ID=w295, data in=w285, error in (no error)=w292, 9:-1 ("timeout ms (25000)")) -> (connection ID out=w294:refnum<k5>, bytes written=→"bytes written 12":i32, error out=w291:errorcluster)
    n258 = Wait (ms)(milliseconds to wait=u32 1000) -> ()  [unwired: 1 out]
  }
  n259 = while {
    tunnel: w26 -> [w301]
    tunnel: [w299] -> w25
    stop <- w298 stop-if-true
    n260 = event shown="[0] \"\": Value Change" {
      selector: _ -> [_ _]
      dyn-events: _ -> [_ _]
      timeout: _ -> [_ _]
      tunnel: [w305 _] -> w300
      tunnel: [_ FALSE] -> w298
      event Value Change {
        n261 = event-data() -> ()  [unwired: 1 in, 6 out]
        n262 = Type Cast(x="?") -> (*(type *) &x=w306:string)  [unwired: 1 in]
        n263 = Number To Decimal String(number=1) -> (decimal integer string=w307:string)  [unwired: 1 in]
        n264 = Concatenate Strings(w307, w306) -> (w305:string)
        "?" <- "?"
      }
      event Timeout {
        n265 = event-data() -> ()  [unwired: 1 in, 3 out]
      }
    }
    n266 = String Length(string=w300) -> (length=w303:i32)
    n267 = Type Cast(x=w303) -> (*(type *) &x=w302:string)  [unwired: 1 in]
    n268 = TCP Write(connection ID=w301, data in=w302) -> (error out=w297:errorcluster)  [unwired: 2 in, 2 out]
    n269 = TCP Write(connection ID=w301, data in=w300, error in (no error)=w297) -> (connection ID out=w299:refnum<k5>)  [unwired: 1 in, 2 out]
  }
  n270 = while {
    shift-right: [w324] -> w22
    shift-left: w21 -> [w326]
    shift-right: [w321] -> w24
    shift-left: w23 -> [w323]
    stop <- "stop 6" stop-if-true
    n271 = local read item#46() -> (w311:dbl)
    n272 = Format Into String(w311) -> (resulting string=w315:string)  [unwired: 3 in, 1 out]
    n273 = String Length(string=w315) -> (length=w314:i32)
    n274 = Format Into String(w314) -> (resulting string=w313:string)  [unwired: 3 in, 1 out]
    n275 = TCP Write(connection ID=w326, data in=w313, error in (no error)=w323, 9:-1 ("timeout ms (25000)")) -> (connection ID out=w325:refnum<k5>, bytes written=→"bytes written 7":i32, error out=w322:errorcluster)
    n276 = case shown="\"Low\", Default" "?" {
      frame "Low", Default {
        n277 = local write item#46(20.0 ("Thermometer")) -> ()
      }
      frame "Medium" {
        n278 = local write item#46(40.0 ("Thermometer")) -> ()
      }
      frame "High" {
        n279 = local write item#46(60.0 ("Thermometer")) -> ()
      }
    }
    n280 = TCP Write(connection ID=w325, data in=w315, error in (no error)=w322, 9:-1 ("timeout ms (25000)")) -> (connection ID out=w324:refnum<k5>, bytes written=→"bytes written 8":i32, error out=w321:errorcluster)
    n281 = Wait (ms)(milliseconds to wait=u32 1000) -> ()  [unwired: 1 out]
  }
  n282 = while {
    shift-right: [w344] -> w16
    shift-left: w15 -> [w346]
    shift-right: [w341] -> w18
    shift-left: w17 -> [w343]
    stop <- "stop 7" stop-if-true
    n283 = local read item#51() -> (w331:dbl)
    n284 = Format Into String(w331) -> (resulting string=w335:string)  [unwired: 3 in, 1 out]
    n285 = String Length(string=w335) -> (length=w334:i32)
    n286 = Format Into String(w334) -> (resulting string=w333:string)  [unwired: 3 in, 1 out]
    n287 = TCP Write(connection ID=w346, data in=w333, error in (no error)=w343, 9:-1 ("timeout ms (25000)")) -> (connection ID out=w345:refnum<k5>, bytes written=→"bytes written 9":i32, error out=w342:errorcluster)
    n288 = case shown="\"Default\"" "?" {
      frame "Cold", Default {
        n289 = local write item#51(20.0 ("Thermometer")) -> ()
      }
      frame "Default" {
        n290 = local write item#51(40.0 ("Thermometer")) -> ()
      }
      frame "Hot" {
        n291 = local write item#51(60.0 ("Thermometer")) -> ()
      }
    }
    n292 = TCP Write(connection ID=w345, data in=w335, error in (no error)=w342, 9:-1 ("timeout ms (25000)")) -> (connection ID out=w344:refnum<k5>, bytes written=→"bytes written 10":i32, error out=w341:errorcluster)
    n293 = Wait (ms)(milliseconds to wait=u32 1000) -> ()  [unwired: 1 out]
  }
  n294 = property on="stop 9" class="Bool"("Visible"=FALSE) -> ()  [unwired: 2 in, 2 out]
  n295 = TCP Close Connection(connection ID=w25) -> ()  [unwired: 2 in, 2 out]
  n296 = TCP Close Connection(connection ID=w10, error in (no error)=w12) -> ()  [unwired: 1 in, 2 out]
  n297 = TCP Close Connection(connection ID=w22, error in (no error)=w24) -> ()  [unwired: 1 in, 2 out]
  n298 = TCP Close Connection(connection ID=w16, error in (no error)=w18) -> ()  [unwired: 1 in, 2 out]
  n299 = while {
    stop <- "stop 5" stop-if-true
    n300 = local read item#33() -> (w354:bool)
    n301 = And(x=w354, y="?") -> (x .and. y?=w350:bool)
    n302 = case shown="\"Rinse\"" "?" {
      tunnel: w350 -> [w355 w377 w399 w421]
      frame "Soak" {
        n303 = case shown="True" w355 {
          frame False {
            w359 = 0
            n304 = property class="Enum (strict)"("DisabledEnum"=w359) -> ()  [unwired: 2 in, 2 out]
            n305 = property class="Slide (strict)"("DisabledEnum"=w359) -> ()  [unwired: 2 in, 2 out]
            n306 = property class="Slide (strict)"("DisabledEnum"=w359) -> ()  [unwired: 2 in, 2 out]
            n307 = flat-sequence {
              frame #0 {
                n308 = local write item#36("Stand by") -> ()
              }
            }
          }
          frame True {
            w363 = 1
            n309 = flat-sequence {
              frame #0 {
                n310 = local read item#34() -> (w365:dbl)
                n311 = Greater Than 0?(x=w365) -> (x > 0?=w364:bool)
                n312 = case shown="True" w364 {
                  frame False {
                  }
                  frame True {
                    n313 = local read item#34() -> (w368:dbl)
                    n314 = Multiply(x=1000, y=w368) -> (x*y=w367:dbl)
                    n315 = Wait (ms)(milliseconds to wait=w367) -> ()  [unwired: 1 out]
                    n316 = local write item#36("Soak") -> ()
                  }
                }
              }
            }
            n317 = property class="Enum (strict)"("DisabledEnum"=w363) -> ()  [unwired: 2 in, 2 out]
            n318 = property class="Slide (strict)"("DisabledEnum"=w363) -> ()  [unwired: 2 in, 2 out]
            n319 = property class="Slide (strict)"("DisabledEnum"=w363) -> ()  [unwired: 2 in, 2 out]
            n320 = local read item#34() -> (w362:dbl)
            n321 = Not Equal To 0?(x=w362) -> (x != 0?=w361:bool)
            n322 = case shown="True" w361 {
              frame False {
              }
              frame True {
                n323 = local read item#34() -> (w370:dbl)
                n324 = for {
                  N: w370 -> [w376]
                  i -> [w372]
                  stop <- "stop default true 5" stop-if-true
                  n325 = Increment(x=w372) -> (x+1=w375:i32)
                  n326 = Wait (ms)(milliseconds to wait=u32 1000) -> ()  [unwired: 1 out]
                  n327 = Subtract(x=w376, y=w375) -> (x-y=w373:i32)
                  n328 = local write item#34(w373) -> ()
                }
              }
            }
          }
        }
        n329 = local read item#34() -> (w357:dbl)
        n330 = Greater Or Equal To 0?(x=w357) -> (x >= 0?=w356:bool)
        n331 = case shown="True" w356 {
          frame False {
          }
          frame True {
            n332 = local read item#37() -> (w358:dbl)
            n333 = local write item#34(w358) -> ()
          }
        }
      }
      frame "Wash" {
        n334 = local read item#34() -> (w379:dbl)
        n335 = Equal To 0?(x=w379) -> (x = 0?=w378:bool)
        n336 = case shown="True" w378 {
          frame False {
          }
          frame True {
            n337 = local read item#37() -> (w380:dbl)
            n338 = local write item#34(w380) -> ()
          }
        }
        n339 = case shown="False" w377 {
          frame False {
            w381 = 0
            n340 = property class="Enum (strict)"("DisabledEnum"=w381) -> ()  [unwired: 2 in, 2 out]
            n341 = property class="Slide (strict)"("DisabledEnum"=w381) -> ()  [unwired: 2 in, 2 out]
            n342 = property class="Slide (strict)"("DisabledEnum"=w381) -> ()  [unwired: 2 in, 2 out]
            n343 = flat-sequence {
              frame #0 {
                n344 = local write item#36("Stand by") -> ()
              }
            }
          }
          frame True {
            w385 = 1
            n345 = flat-sequence {
              frame #0 {
                n346 = local read item#34() -> (w387:dbl)
                n347 = Greater Than 0?(x=w387) -> (x > 0?=w386:bool)
                n348 = case shown="True" w386 {
                  frame False {
                  }
                  frame True {
                    n349 = local read item#34() -> (w390:dbl)
                    n350 = Multiply(x=1000, y=w390) -> (x*y=w389:dbl)
                    n351 = Wait (ms)(milliseconds to wait=w389) -> ()  [unwired: 1 out]
                    n352 = local write item#36("Wash") -> ()
                  }
                }
              }
            }
            n353 = property class="Enum (strict)"("DisabledEnum"=w385) -> ()  [unwired: 2 in, 2 out]
            n354 = property class="Slide (strict)"("DisabledEnum"=w385) -> ()  [unwired: 2 in, 2 out]
            n355 = property class="Slide (strict)"("DisabledEnum"=w385) -> ()  [unwired: 2 in, 2 out]
            n356 = local read item#34() -> (w384:dbl)
            n357 = Not Equal To 0?(x=w384) -> (x != 0?=w383:bool)
            n358 = case shown="True" w383 {
              frame False {
              }
              frame True {
                n359 = local read item#34() -> (w392:dbl)
                n360 = for {
                  N: w392 -> [w398]
                  i -> [w394]
                  stop <- "stop default true 6" stop-if-true
                  n361 = Increment(x=w394) -> (x+1=w397:i32)
                  n362 = Wait (ms)(milliseconds to wait=u32 1000) -> ()  [unwired: 1 out]
                  n363 = Subtract(x=w398, y=w397) -> (x-y=w395:i32)
                  n364 = local write item#34(w395) -> ()
                }
              }
            }
          }
        }
      }
      frame "Rinse" {
        n365 = local read item#34() -> (w401:dbl)
        n366 = Greater Or Equal To 0?(x=w401) -> (x >= 0?=w400:bool)
        n367 = case shown="True" w400 {
          frame False {
          }
          frame True {
            n368 = local read item#37() -> (w402:dbl)
            n369 = local write item#34(w402) -> ()
          }
        }
        n370 = case shown="True" w399 {
          frame False {
            w403 = 0
            n371 = property class="Slide (strict)"("DisabledEnum"=w403) -> ()  [unwired: 2 in, 2 out]
            n372 = property class="Slide (strict)"("DisabledEnum"=w403) -> ()  [unwired: 2 in, 2 out]
            n373 = property class="Enum (strict)"("DisabledEnum"=w403) -> ()  [unwired: 2 in, 2 out]
            n374 = flat-sequence {
              frame #0 {
                n375 = local write item#36("Stand by") -> ()
              }
            }
          }
          frame True {
            w407 = 1
            n376 = flat-sequence {
              frame #0 {
                n377 = local read item#34() -> (w409:dbl)
                n378 = Greater Than 0?(x=w409) -> (x > 0?=w408:bool)
                n379 = case shown="True" w408 {
                  frame False {
                  }
                  frame True {
                    n380 = local read item#34() -> (w412:dbl)
                    n381 = Multiply(x=1000, y=w412) -> (x*y=w411:dbl)
                    n382 = Wait (ms)(milliseconds to wait=w411) -> ()  [unwired: 1 out]
                    n383 = local write item#36("Rinse") -> ()
                  }
                }
              }
            }
            n384 = property class="Enum (strict)"("DisabledEnum"=w407) -> ()  [unwired: 2 in, 2 out]
            n385 = property class="Slide (strict)"("DisabledEnum"=w407) -> ()  [unwired: 2 in, 2 out]
            n386 = property class="Slide (strict)"("DisabledEnum"=w407) -> ()  [unwired: 2 in, 2 out]
            n387 = local read item#34() -> (w406:dbl)
            n388 = Not Equal To 0?(x=w406) -> (x != 0?=w405:bool)
            n389 = case shown="True" w405 {
              frame False {
              }
              frame True {
                n390 = local read item#34() -> (w414:dbl)
                n391 = for {
                  N: w414 -> [w420]
                  i -> [w416]
                  stop <- "stop default true 7" stop-if-true
                  n392 = Increment(x=w416) -> (x+1=w419:i32)
                  n393 = Wait (ms)(milliseconds to wait=u32 1000) -> ()  [unwired: 1 out]
                  n394 = Subtract(x=w420, y=w419) -> (x-y=w417:i32)
                  n395 = local write item#34(w417) -> ()
                }
              }
            }
          }
        }
      }
      frame "Spin" {
        n396 = local read item#34() -> (w422:dbl)
        n397 = Greater Or Equal To 0?(x=w422) -> (x >= 0?=w423:bool)
        n398 = case shown="True" w423 {
          frame False {
          }
          frame True {
            n399 = local read item#37() -> (w424:dbl)
            n400 = local write item#34(w424) -> ()
          }
        }
        n401 = case shown="False" w421 {
          frame False {
            w425 = 0
            n402 = property class="Enum (strict)"("DisabledEnum"=w425) -> ()  [unwired: 2 in, 2 out]
            n403 = property class="Slide (strict)"("DisabledEnum"=w425) -> ()  [unwired: 2 in, 2 out]
            n404 = property class="Slide (strict)"("DisabledEnum"=w425) -> ()  [unwired: 2 in, 2 out]
            n405 = flat-sequence {
              frame #0 {
                n406 = local write item#36("Stand by") -> ()
              }
            }
          }
          frame True {
            w429 = 1
            n407 = flat-sequence {
              frame #0 {
                n408 = local read item#34() -> (w431:dbl)
                n409 = Greater Than 0?(x=w431) -> (x > 0?=w430:bool)
                n410 = case shown="True" w430 {
                  frame False {
                  }
                  frame True {
                    n411 = local read item#34() -> (w434:dbl)
                    n412 = Multiply(x=1000, y=w434) -> (x*y=w433:dbl)
                    n413 = Wait (ms)(milliseconds to wait=w433) -> ()  [unwired: 1 out]
                    n414 = local write item#36("Spin") -> ()
                  }
                }
              }
            }
            n415 = property class="Enum (strict)"("DisabledEnum"=w429) -> ()  [unwired: 2 in, 2 out]
            n416 = property class="Slide (strict)"("DisabledEnum"=w429) -> ()  [unwired: 2 in, 2 out]
            n417 = property class="Slide (strict)"("DisabledEnum"=w429) -> ()  [unwired: 2 in, 2 out]
            n418 = local read item#34() -> (w428:dbl)
            n419 = Not Equal To 0?(x=w428) -> (x != 0?=w427:bool)
            n420 = case shown="True" w427 {
              frame False {
              }
              frame True {
                n421 = local read item#34() -> (w436:dbl)
                n422 = for {
                  N: w436 -> [w442]
                  i -> [w438]
                  stop <- "stop default true 8" stop-if-true
                  n423 = Increment(x=w438) -> (x+1=w441:i32)
                  n424 = Wait (ms)(milliseconds to wait=u32 1000) -> ()  [unwired: 1 out]
                  n425 = Subtract(x=w442, y=w441) -> (x-y=w439:i32)
                  n426 = local write item#34(w439) -> ()
                }
              }
            }
          }
        }
      }
    }
  }
  n427 = TCP Open Connection(remote port or service name=696969, timeout ms (60000)=60000) -> (connection ID=w3:refnum<k5>)  [unwired: 3 in, 1 out]
  n428 = while {
    tunnel: [w446] -> w6
    tunnel: w3 -> [w445]
    stop <- FALSE stop-if-true
    n429 = local read item#36() -> (w444:string)
    n430 = Type Cast(x=w444) -> (*(type *) &x=w443:string)  [unwired: 1 in]
    n431 = String Length(string=w443) -> (length=w450:i32)
    n432 = Type Cast(x=w450) -> (*(type *) &x=w449:string)  [unwired: 1 in]
    n433 = TCP Write(connection ID=w445, data in=w449) -> (connection ID out=w447:refnum<k5>)  [unwired: 2 in, 2 out]
    n434 = TCP Write(connection ID=w447, data in=w443) -> (connection ID out=w446:refnum<k5>)  [unwired: 2 in, 2 out]
  }
  n435 = TCP Close Connection(connection ID=w6) -> ()  [unwired: 2 in, 2 out]
